vi "send_trajectory.vi"(0 "simx in":T1={"Config"={"Trajectory"={"Number of frames"=0, "Frame number"=0, "Trajectory"=""}, "Weather"={"id"=""}}, "Connections"={"Simulator Connection"=refnum, "server_ip"="127.0.0.1", "Port"=0, "Sensor connections"=[]}, "Map"={"lanes"={"x"=[], "y"=[], "z"=[]}, "StartPosition"={"start_points"={"locations"=[], "rotations"=[], "type"=[]}, "StartRotation"=[], "StartLocation"=[]}, "Draw Map Size"={"Width"=0, "Height"=0}, "DrawArea"={"min_Y"=0.0, "min_X"=0.0, "Scale X"=0.0, "Scale Y"=0.0}, "Map"=bytes[0], "Map Geojson"=""}}, 2 "Trajectory Configuration":path, 5 "error in":errorcluster) -> (6 "simx out":T1={"Config"={"Trajectory"={"Number of frames"=0, "Frame number"=0, "Trajectory"=""}, "Weather"={"id"=""}}, "Connections"={"Simulator Connection"=refnum, "server_ip"="127.0.0.1", "Port"=0, "Sensor connections"=[]}, "Map"={"lanes"={"x"=[], "y"=[], "z"=[]}, "StartPosition"={"start_points"={"locations"=[], "rotations"=[], "type"=[]}, "StartRotation"=[], "StartLocation"=[]}, "Draw Map Size"={"Width"=0, "Height"=0}, "DrawArea"={"min_Y"=0.0, "min_X"=0.0, "Scale X"=0.0, "Scale Y"=0.0}, "Map"=bytes[0], "Map Geojson"=""}}, 7 "Trajectory configuration":string, 8 "error out":errorcluster)   [LabVIEW 2019, in "Lib_Simx.lvlib"]
doc: "Reads a trajectory file and sends it to the server."
uses:
  Lib_Simx.lvlib
  controls/simx_connection.ctl
  controls/config.ctl
  controls/trajectory.ctl
  controls/weather.ctl
  controls/connections.ctl
  controls/start_points.ctl
  <vilib>/Utility/miscctls.llb/LVBoundsTypeDef.ctl
  tools/simx_common.vi
panel:
  out "Response":string
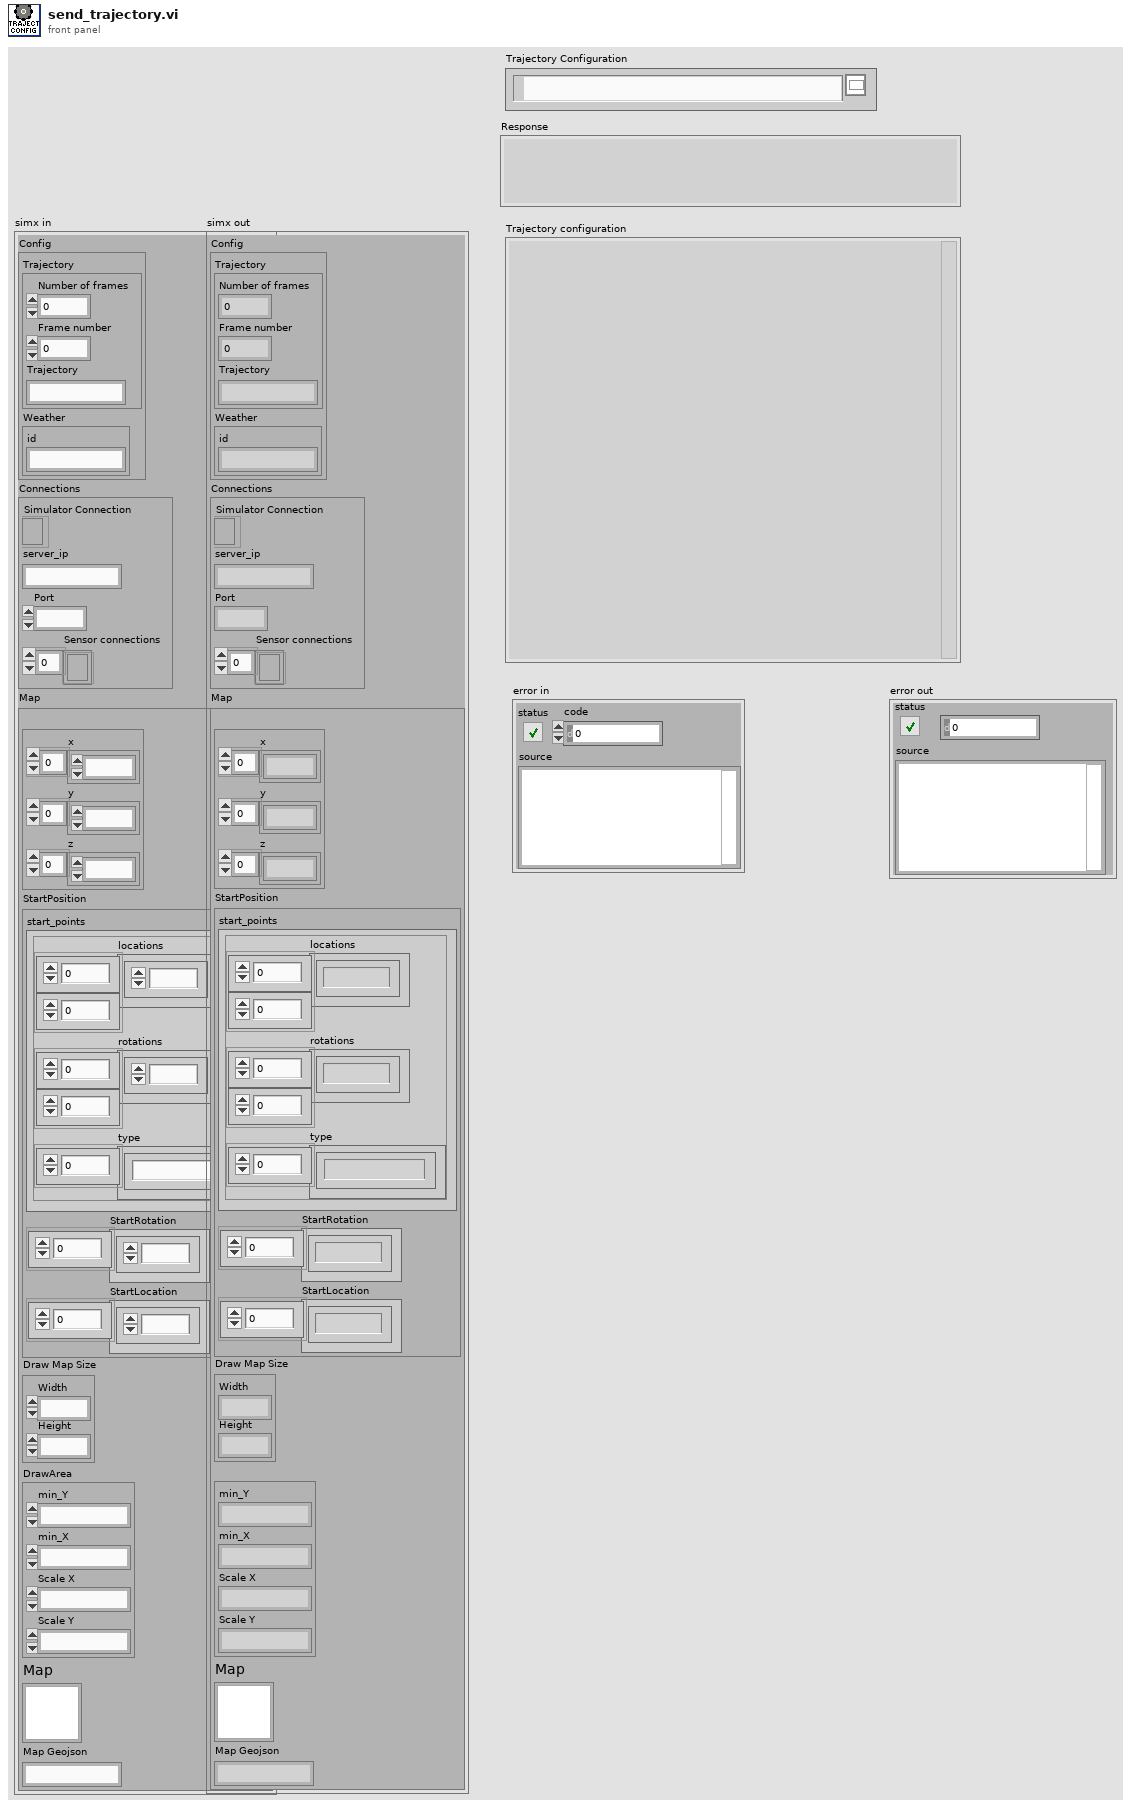
[diagram p1: front panel]
types:
  T1 = typedef "Lib_Simx.lvlib/simx_connection.ctl" = cluster{"Config":T2, "Connections":T5, "Map":cluster{"lanes":cluster{"x":dbl[], "y":dbl[], "z":dbl[]}, "StartPosition":cluster{"start_points":T6, "StartRotation":dbl[], "StartLocation":dbl[]}, "Draw Map Size":T7, "DrawArea":cluster{"min_Y":dbl, "min_X":dbl, "Scale X":dbl, "Scale Y":dbl}, "Map":picture, "Map Geojson":string}}
  T2 = typedef "Lib_Simx.lvlib/config.ctl" = cluster{"Trajectory":T3, "Weather":T4}
  T3 = typedef "Lib_Simx.lvlib/trajectory.ctl" = cluster{"Number of frames":i32, "Frame number":i32, "Trajectory":string}
  T4 = typedef "Lib_Simx.lvlib/weather.ctl" = cluster{"id":string}
  T5 = typedef "Lib_Simx.lvlib/connections.ctl" = cluster{"Simulator Connection":refnum<k5>, "server_ip":string, "Port":i32, "Sensor connections":refnum<k5>[]}
  T6 = typedef "Lib_Simx.lvlib/start_points.ctl" = cluster{"locations":dbl[][], "rotations":dbl[][], "type":string[]}
  T7 = typedef "LVBoundsTypeDef.ctl" = cluster{"Width":u32, "Height":u32}
  T8 = cluster{"game_time":dbl, "time":dbl, "frame":cluster{"velocity":dbl[], "tags":string[], "position":dbl[], "angular_velocity":dbl[], "name":string, "wheel_speed":dbl[], "wheels":cluster{"id":i32, "orientation":dbl[]}[], "orientation":cluster{"yaw":dbl, "pitch":dbl, "roll":dbl}}[]}[]
  T9 = cluster{"game_time":dbl, "time":dbl, "frame":cluster{"velocity":dbl[], "tags":string[], "position":dbl[], "angular_velocity":dbl[], "name":string, "wheel_speed":dbl[], "wheels":cluster{"id":i32, "orientation":dbl[]}[], "orientation":cluster{"yaw":dbl, "pitch":dbl, "roll":dbl}}[]}
  T10 = cluster{"velocity":dbl[], "tags":string[], "position":dbl[], "angular_velocity":dbl[], "name":string, "wheel_speed":dbl[], "wheels":cluster{"id":i32, "orientation":dbl[]}[], "orientation":cluster{"yaw":dbl, "pitch":dbl, "roll":dbl}}[]
  T11 = cluster{"velocity":dbl[], "tags":string[], "position":dbl[], "angular_velocity":dbl[], "name":string, "wheel_speed":dbl[], "wheels":cluster{"id":i32, "orientation":dbl[]}[], "orientation":cluster{"yaw":dbl, "pitch":dbl, "roll":dbl}}
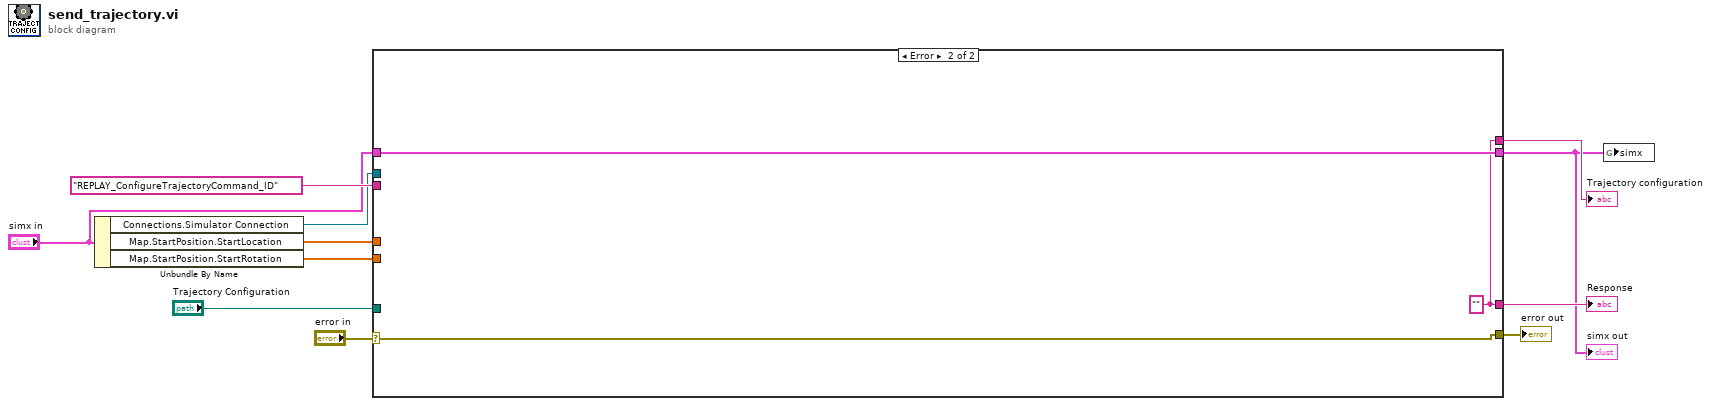
[diagram p0: block diagram]
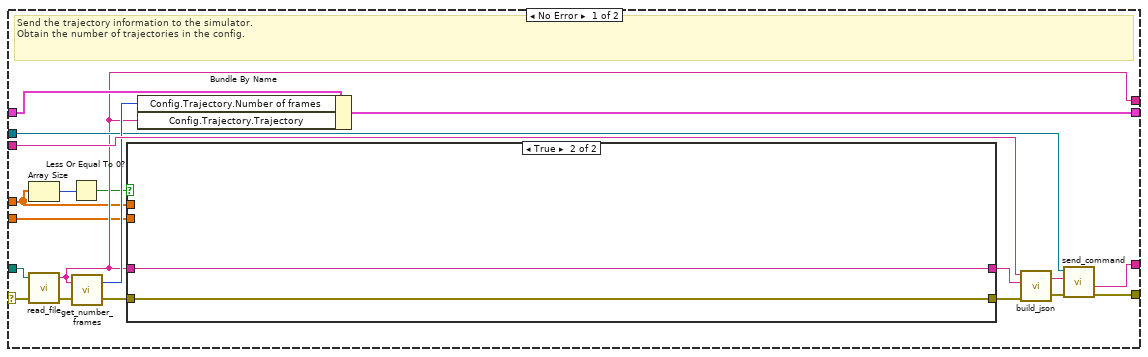
[diagram p2: hidden frame]
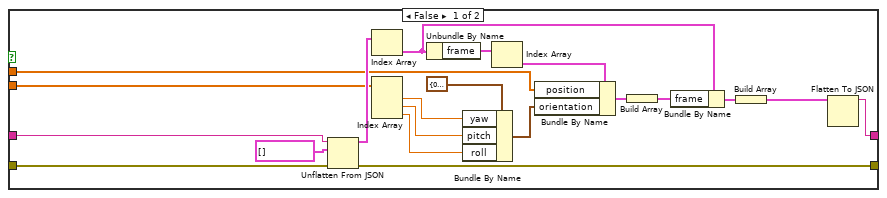
[diagram p3: hidden frame]
diagram:
  n1 = Unbundle By Name("simx in") -> ("Connections.Simulator Connection"=w6:refnum<k5>, "Map.StartPosition.StartLocation"=w3:dbl[], "Map.StartPosition.StartRotation"=w2:dbl[])
  n2 = case shown="Error" "error in" {
    selector: "error in" -> [w20 w56]
    tunnel: [w31 w54] -> w11
    tunnel: [w29 w56] -> w10
    tunnel: "REPLAY_ConfigureTrajectoryCommand_ID" ("Command_ID") -> [w30 _]
    tunnel: "simx in" -> [w24 w55]
    tunnel: [w25 w55] -> w1
    tunnel: w6 -> [w23 _]
    tunnel: [w19 w54] -> w5
    tunnel: "Trajectory Configuration" -> [w22 _]
    tunnel: w3 -> [w18 _]
    tunnel: w2 -> [w15 _]
    frame No Error {
      # "Send the trajectory information to the simulator. \nObtain the number of trajectories in the config."
      n3 = Array Size(array=w18) -> (size(s)=w17:i32)
      n4 = call "read_file.vi"("error in"=w20, "File path in"=w22) -> ("error out"=w21:errorcluster, "Trajectory or Scenario read"=w19:string)  [unwired: 1 in, 1 out]
      n5 = Less Or Equal To 0?(x=w17) -> (x <= 0?=w16:bool)
      n6 = call "get_number_frames.vi"("error in"=w21, "Trajectory (JSON)"=w19) -> ("error out"=w13:errorcluster, "Number of frames"=w26:i32)
      n7 = case shown="True" w16 {
        tunnel: w19 -> [w42 w53]
        tunnel: [w41 w53] -> w14
        tunnel: w18 -> [w40 _]
        tunnel: w15 -> [w37 _]
        tunnel: w13 -> [w33 w52]
        tunnel: [w32 w52] -> w12
        frame False {
          n8 = Unflatten From JSON(JSON string=w42, type and defaults=T8 [], error in (no error)=w33) -> (value=w50:T8, error out=w32:errorcluster)  [unwired: 4 in]
          n9 = Index Array(array=w50) -> (element=w46:T9)  [unwired: 1 in]
          n10 = Index Array(array=w37) -> (element #1=w36:dbl, element #2=w35:dbl, element #3=w34:dbl)  [unwired: 3 in]
          n11 = Unbundle By Name(w46) -> ("frame"=w49:T10)
          n12 = Bundle By Name(cluster=cluster{"yaw":dbl, "pitch":dbl, "roll":dbl} {"yaw"=0.0, "pitch"=0.0, "roll"=0.0} ("orientation"), "yaw"=w36, "pitch"=w35, "roll"=w34) -> (w38:cluster{"yaw":dbl, "pitch":dbl, "roll":dbl})
          n13 = Index Array(array=w49) -> (element=w48:T11)  [unwired: 1 in]
          n14 = Bundle By Name(cluster=w48, "position"=w40, "orientation"=w38) -> (w47:T11)
          n15 = Build Array(w47) -> (w45:T10)
          n16 = Bundle By Name(cluster=w46, "frame"=w45) -> (w44:T9)
          n17 = Build Array(w44) -> (w43:T8)
          n18 = Flatten To JSON(anything=w43) -> (JSON string=w41:string)  [unwired: 2 in, 1 out]
        }
        frame True {
        }
      }
      n19 = Bundle By Name(cluster=w24, "Config.Trajectory.Number of frames"=w26, "Config.Trajectory.Trajectory"=w19) -> (w25:T1)
      n20 = call "build_json.vi"("error in"=w12, "Message"=w14, "Command_ID"=w30) -> ("error out"=w27:errorcluster, "JSON Out"=w28:string)  [unwired: 1 in]
      n21 = call "send_command.vi"("error in"=w27, "JSON Command"=w28, "TCP Network Connection in"=w23) -> ("error out"=w29:errorcluster, "Response"=w31:string)  [unwired: 1 in, 2 out]
    }
    frame Error {
      w54 = "" ("response")
    }
  }
  "Response" <- w11
  "error out" <- w10
  "simx out" <- w1
  "Trajectory configuration" <- w5
  n22 = global write "simx_common.vi" "simx"(w1) -> ()
